vi "close camera.vi"(8 "error in (no error)":errorcluster, 11 "Camera":T1) -> (0 "error out":errorcluster, 3 "Camera out":T1)   [LabVIEW 2024, in "Vision.lvlib"]
uses:
  Vision.lvlib
  camera.ctl
  camera driver.ctl
  <vilib>/userDefined/High Color/IMAQdx.ctl
  C:/Users/cfang/Desktop/nebraska-silicon-lab/pixel-gantry-control/Gantry/Shared Components/bin.bak/uEyeDotNet.dll
  bin.bak/uEyeDotNet.dll
  <vilib>/vision/driver/NI_Vision_Acquisition_Software.lvlib
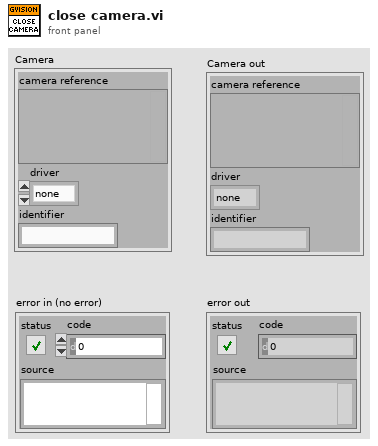
[diagram p1: front panel]
types:
  T1 = typedef "Vision.lvlib/camera.ctl" = cluster{"camera reference":variant, "driver":T2, "identifier":string}
  T2 = typedef "Vision.lvlib/camera driver.ctl" = enum16{"none", "ueye", "wmf", "imaqdx"}
  T3 = typedef "IMAQdx.ctl" = refnum<k21>
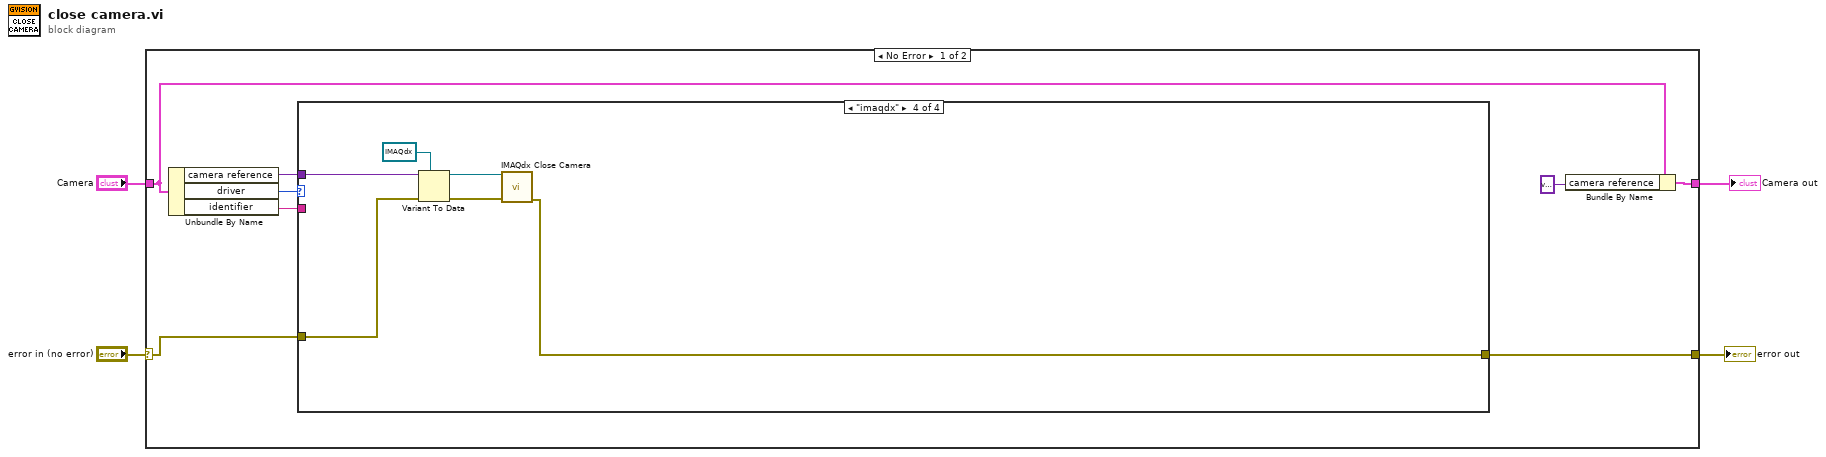
[diagram p0: block diagram]
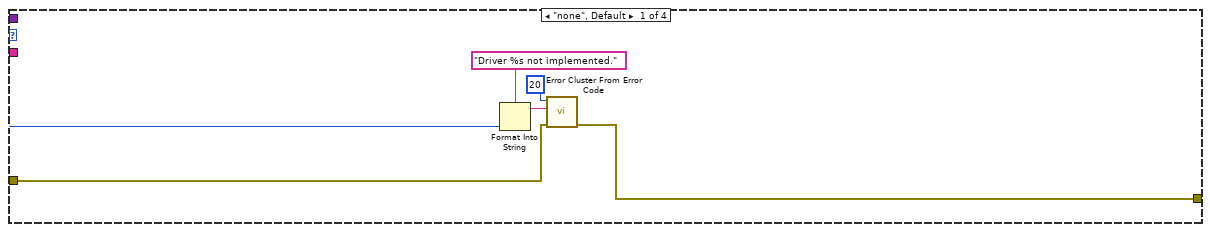
[diagram p2: hidden frame]
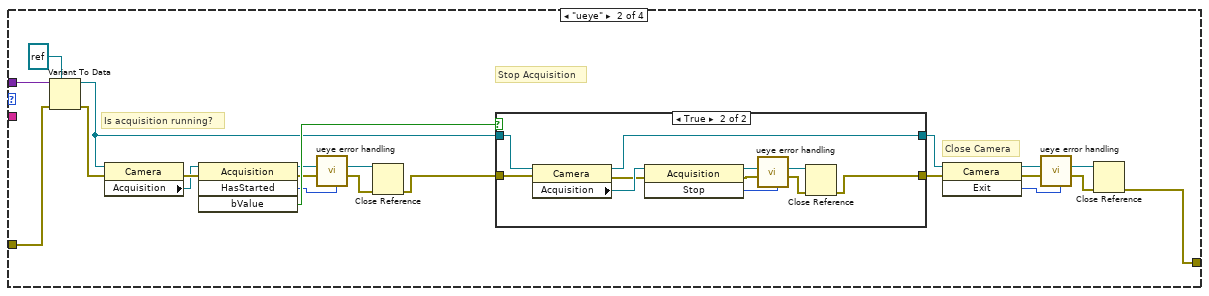
[diagram p3: hidden frame]
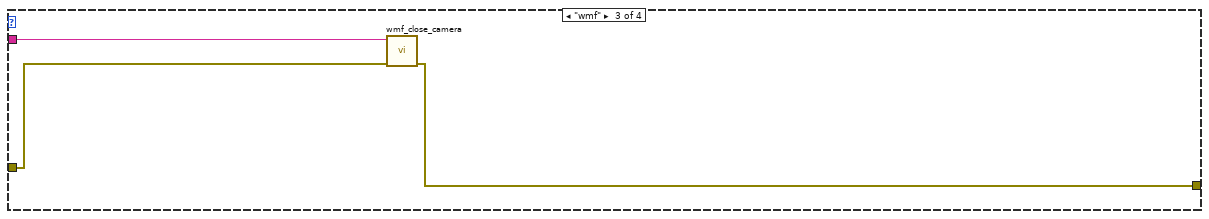
[diagram p5: hidden frame]
diagram:
  n1 = case shown="No Error" "error in (no error)" {
    selector: "error in (no error)" -> [w12 w61]
    tunnel: [w9 w61] -> w3
    tunnel: "Camera" -> [w8 w60]
    tunnel: [w6 w60] -> w1
    frame No Error {
      n2 = Unbundle By Name(w8) -> ("camera reference"=w10:variant, "driver"=w11:T2, "identifier"=w5:string)
      n3 = case shown="\"imaqdx\"" w11 {
        selector: w11 -> [w15 _ _ _]
        tunnel: w12 -> [w17 w33 w52 w57]
        tunnel: w10 -> [_ w37 _ w58]
        tunnel: [w13 w19 w51 w54] -> w9
        tunnel: w5 -> [_ _ w53 _]
        frame "none", Default {
          n4 = Format Into String(format string="Driver %s not implemented.", w15) -> (resulting string=w14:string)  [unwired: 2 in, 1 out]
          n5 = call <vilib>:"Error Cluster From Error Code.vi"("error in (no error)"=w17, "error message (\"\")"=w14, "error code (0)"=20) -> ("error out"=w13:errorcluster)  [unwired: 6 in]
        }
        frame "ueye" {
          # "Close Camera"
          # "Is acquisition running?"
          # "Stop Acquisition"
          n6 = Variant To Data(error in=w33, type=refnum<k24> refnum ("reference"), Variant=w37) -> (data=w31:refnum<k24>, error out=w32:errorcluster)
          n7 = property class="Camera"(reference=w31, error in=w32) -> (error out=w36:errorcluster, "Acquisition"=w35:refnum<k24>)  [unwired: 1 out]
          n8 = invoke class="Acquisition" method="HasStarted"(reference=w35, error in=w36) -> (reference out=w24:refnum<k24>, error out=w28:errorcluster, "HasStarted"=w27:i32, "bValue"=w34:bool)  [unwired: 2 in]
          n9 = call "ueye error handling.vi"("Error Code"=w27, "reference in"=w24, "Error In"=w28) -> ("Error Out"=w23:errorcluster)  [unwired: 8 in]
          n10 = Close Reference(reference=w24, error in (no error)=w23) -> (error out=w22:errorcluster)
          n11 = case shown="True" w34 {
            tunnel: [w40 w43] -> w29
            tunnel: w22 -> [w40 w50]
            tunnel: w31 -> [w39 w42]
            tunnel: [w39 w41] -> w30
            frame False {
            }
            frame True {
              n12 = property class="Camera"(reference=w42, error in=w50) -> (reference out=w41:refnum<k24>, error out=w48:errorcluster, "Acquisition"=w49:refnum<k24>)
              n13 = invoke class="Acquisition" method="Stop"(reference=w49, error in=w48) -> (reference out=w45:refnum<k24>, error out=w47:errorcluster, "Stop"=w46:i32)  [unwired: 1 in]
              n14 = call "ueye error handling.vi"("Error Code"=w46, "reference in"=w45, "Error In"=w47) -> ("Error Out"=w44:errorcluster)  [unwired: 8 in]
              n15 = Close Reference(reference=w45, error in (no error)=w44) -> (error out=w43:errorcluster)
            }
          }
          n16 = invoke class="Camera" method="Exit"(reference=w30, error in=w29) -> (reference out=w20:refnum<k24>, error out=w26:errorcluster, "Exit"=w25:i32)  [unwired: 1 in]
          n17 = call "ueye error handling.vi"("Error Code"=w25, "reference in"=w20, "Error In"=w26) -> ("Error Out"=w21:errorcluster)  [unwired: 8 in]
          n18 = Close Reference(reference=w20, error in (no error)=w21) -> (error out=w19:errorcluster)
        }
        frame "wmf" {
          n19 = call "wmf_close_camera.vi"("error in (no error)"=w52, "camera_name"=w53) -> ("error out"=w51:errorcluster)  [unwired: 9 in]
        }
        frame "imaqdx" {
          n20 = Variant To Data(error in=w57, type=T3 refnum ("Session In"), Variant=w58) -> (data=w56:T3, error out=w55:errorcluster)
          n21 = call <vilib>:"IMAQdx Close Camera.vi"("error in"=w55, "Session In"=w56) -> ("error out"=w54:errorcluster)  [unwired: 9 in]
        }
      }
      n22 = Bundle By Name(cluster=w8, "camera reference"=variant) -> (w6:T1)
    }
    frame Error {
    }
  }
  "error out" <- w3
  "Camera out" <- w1
